vi "Deadzone.vi"(4 "Deadzone Limit":dbl, 5 "Value In":dbl) -> (1 "Value Out":dbl)   [LabVIEW 2014]
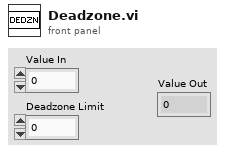
[diagram p1: front panel]
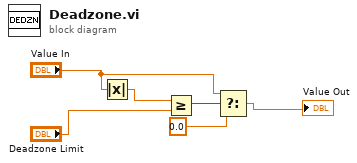
[diagram p0: block diagram]
diagram:
  n1 = Absolute Value(x="Value In") -> (abs(x)=w4:dbl)
  n2 = Greater Or Equal?(x=w4, y="Deadzone Limit") -> (x >= y?=w5:bool)
  n3 = Select(t="Value In", s=w5, f=0.0) -> (s? t:f=→"Value Out":dbl)
